vi "random number array for turning.vi"   [LabVIEW 2016]
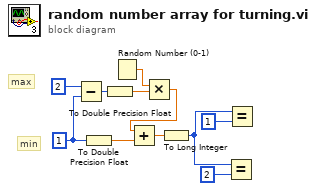
[diagram p0: block diagram]
diagram:
  w9 = 1
  # "min"
  # "max"
  n1 = Subtract(x=2, y=w9) -> (x-y=w10:i32)
  n2 = To Double Precision Float(number=w9) -> (double precision float=w8:dbl)
  n3 = To Double Precision Float(number=w10) -> (double precision float=w7:dbl)
  n4 = Random Number (0-1)() -> (number: 0 to 1=w6:dbl)
  n5 = Multiply(x=w6, y=w7) -> (x*y=w4:dbl)
  n6 = Add(x=w4, y=w8) -> (x+y=w5:dbl)
  n7 = To Long Integer(number=w5) -> (32bit integer=w2:i32)
  n8 = Equal?(x=w2, y=2) -> ()  [unwired: 1 out]
  n9 = Equal?(x=w2, y=1) -> ()  [unwired: 1 out]
